vi "TestExec.Event Counter Log.vi"(5 "Root Name":string="Event Counter", 7 "Log Folder":path, 10 "Reset":bool, 11 "Read(T)/Inc and Save(F)":bool) -> (3 "Event Cnt Out":i32)   [LabVIEW 2019]
uses:
  <vilib>/KATE/Files/File Utils.lvlib
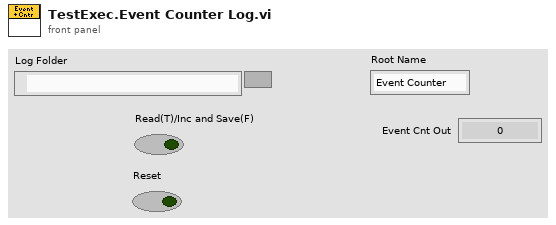
[diagram p1: front panel]
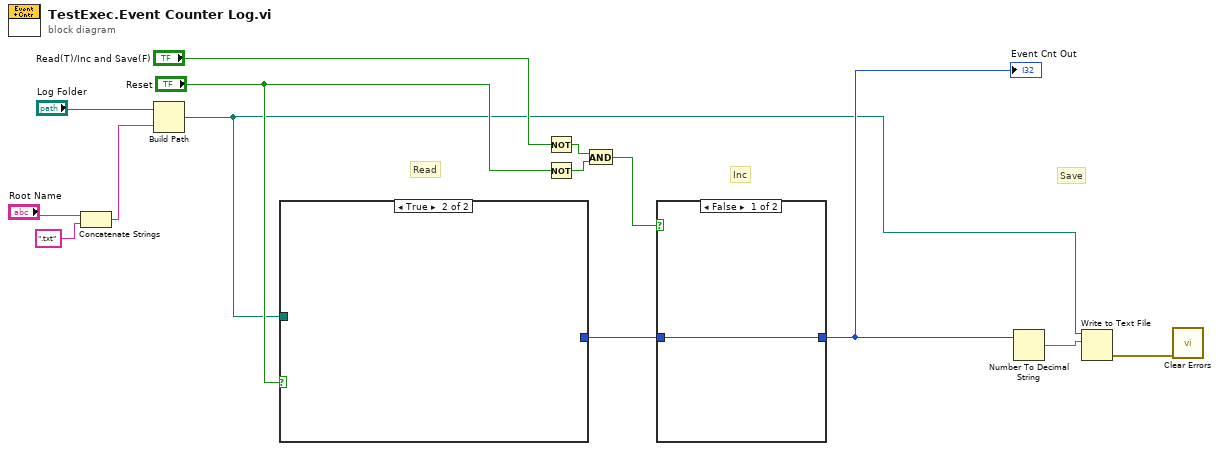
[diagram p0: block diagram]
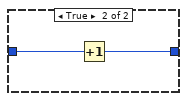
[diagram p2: hidden frame]
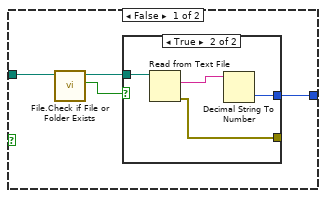
[diagram p3: hidden frame]
diagram:
  # "Save"
  # "Inc"
  # "Read"
  n1 = Concatenate Strings("Root Name", ".txt" ("name or relative path")) -> (w1:string)
  n2 = Build Path(base path="Log Folder", name or relative path=w1) -> (appended path=w5:path)
  n3 = case shown="True" "Reset" {
    tunnel: w5 -> [w18 _]
    tunnel: [w16 _] -> w12
    frame False {
      n4 = call <vilib>:"File.Check if File or Folder Exists.vi"("Path"=w18) -> ("Exists"=w17:bool, "Dup Path"=w15:path)  [unwired: 6 in, 3 out]
      n5 = case shown="True" w17 {
        tunnel: w15 -> [_ w21]
        tunnel: [_ w20] -> w16
        tunnel: [_ w19] -> _
        frame False {
        }
        frame True {
          n6 = Read from Text File(file (use dialog)=w21) -> (text=w22:string, error out=w19:errorcluster)  [unwired: 3 in, 2 out]
          n7 = Decimal String To Number(string=w22) -> (number=w20:i32)  [unwired: 2 in, 1 out]
        }
      }
    }
    frame True {
    }
  }
  n8 = Not(x="Read(T)/Inc and Save(F)") -> (.not. x?=w11:bool)
  n9 = Not(x="Reset") -> (.not. x?=w9:bool)
  n10 = And(x=w11, y=w9) -> (x .and. y?=w7:bool)
  n11 = case shown="False" w7 {
    tunnel: w12 -> [w23 w25]
    tunnel: [w23 w24] -> w6
    frame False {
    }
    frame True {
      n12 = Increment(x=w25) -> (x+1=w24:i32)
    }
  }
  "Event Cnt Out" <- w6
  n13 = Number To Decimal String(number=w6) -> (decimal integer string=w13:string)  [unwired: 1 in]
  n14 = Write to Text File(file (use dialog)=w5, text=w13) -> (error out=w4:errorcluster)  [unwired: 2 in, 2 out]
  n15 = call <vilib>:"Clear Errors.vi"("error in (no error)"=w4) -> ()  [unwired: 5 in, 2 out]
